vi "averageSpectra.vi"(11 "multipleSpectra":dbl[][][](array[numeric])) -> (1 "meanSpectrum":dbl[](array[numeric]), 2 "frequencies":dbl[](array[numeric]), 3 "spectraPlots":cluster{"Array":dbl[], "Array":dbl[]}[](array[cluster]))   [LabVIEW 2013]
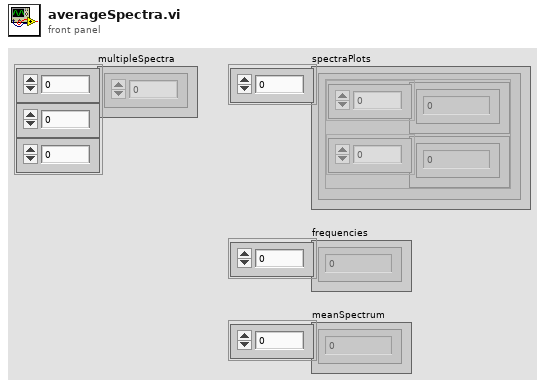
[diagram p1: front panel]
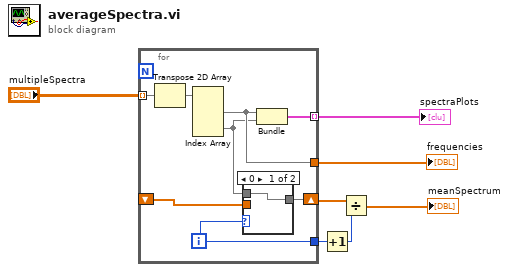
[diagram p0: block diagram]
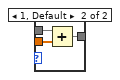
[diagram p2: hidden frame]
diagram:
  n1 = for {
    tunnel: "multipleSpectra" -> [w15] mode=indexing
    tunnel: [w14] -> w3 mode=indexing
    shift-right: [w12] -> w2
    shift-left: _ -> [w11]
    tunnel: [w10] -> w6
    tunnel: [w9] -> w4
    i -> [w9]
    n2 = Transpose 2D Array(2D array=w15) -> (transposed array=w13:dbl[][])
    n3 = Index Array(array=w13) -> (element #1=w10:dbl[], element #2=w8:dbl[])  [unwired: 4 in]
    n4 = case shown="0" w9 {
      tunnel: w8 -> [w16 w19]
      tunnel: [w16 w18] -> w12
      tunnel: w11 -> [_ w17]
      frame 0 {
      }
      frame 1, Default {
        n5 = Add(x=w19, y=w17) -> (x+y=w18:dbl[])
      }
    }
    n6 = Bundle(w10, w8) -> (w14:cluster{dbl[], dbl[]})  [unwired: 1 in]
  }
  "frequencies" <- w6
  "spectraPlots" <- w3
  n7 = Increment(x=w4) -> (x+1=w5:i32)
  n8 = Divide(x=w2, y=w5) -> (x/y=→"meanSpectrum":dbl[])
